vi "Insight_X-axis_OCT.vi"(6 "Index of Refraction":dbl=1.0 format="%_3g", 8 "error in (no error)":errorcluster, 10 "Size of FFT":u32, 11 "Spacing (GHz)":dbl=0.1 format="%_6g") -> (0 "error out":errorcluster, 1 "X-resolution (mm)":dbl, 2 "X-axis":dbl[](array[numeric]))   [LabVIEW 2011]
doc: "Insight Photonic Solutions\n\nThis VI calculates the X-axis for an OCT measurement.\n\nINPUTS\nSize of FFT - This is the size of the two-sided FFT. This may or may not be padded.\nSpacing (GHz) - Optical Frequency Spacing between samples of the measurement.\nIndex of Refraction - Default is 1.\n\nOUTPUTS\nX-resolution - spatial step between points, in millimeters.\nX-axis - Array containing the spatial axis for the OCT measurement.\n\nver 1.0 - original release"
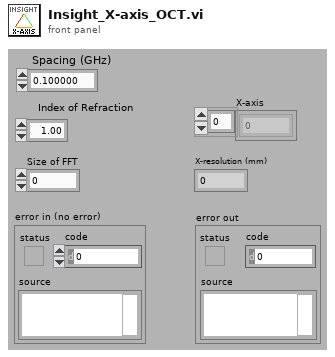
[diagram p1: front panel]
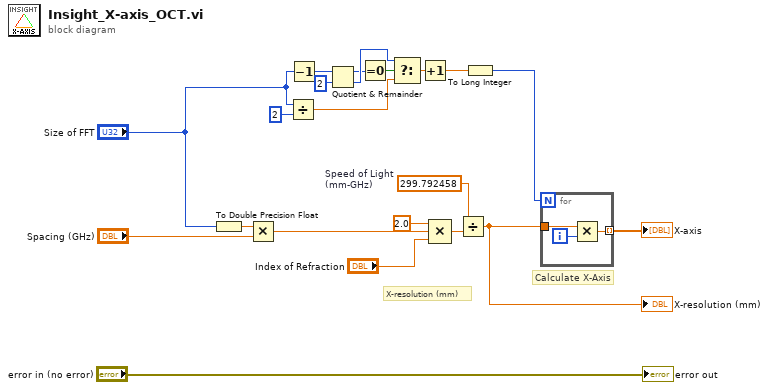
[diagram p0: block diagram]
diagram:
  w17 = 299.792458  # Speed of Light  (mm-GHz)
  # "X-resolution (mm)"
  # "Calculate X-Axis"
  n1 = To Double Precision Float(number="Size of FFT") -> (double precision float=w12:dbl)
  n2 = Multiply(x=w12, y="Spacing (GHz)") -> (x*y=w15:dbl)
  n3 = Divide(x="Size of FFT", y=2) -> (x/y=w11:dbl)
  n4 = Decrement(x="Size of FFT") -> (x-1=w5:u32)
  n5 = Quotient & Remainder(x=w5, y=2) -> (x-y*floor(x/y)=w7:u32, floor(x/y)=w9:u32)
  n6 = Equal To 0?(x=w7) -> (x = 0?=w8:bool)
  n7 = Select(t=w9, s=w8, f=w11) -> (s? t:f=w3:dbl)
  n8 = Increment(x=w3) -> (x+1=w2:dbl)
  n9 = Compound Arithmetic op=MULTIPLY(2.0, w15, "Index of Refraction") -> (w18:dbl)
  n10 = Divide(x=w17, y=w18) -> (x/y=w16:dbl)
  "X-resolution (mm)" <- w16
  n11 = To Long Integer(number=w2) -> (32bit integer=w1:i32)
  n12 = for {
    N: w1 -> [_]
    tunnel: w16 -> [w23]
    tunnel: [w22] -> w14 mode=indexing
    i -> [w24]
    n13 = Multiply(x=w23, y=w24) -> (x*y=w22:dbl)
  }
  "X-axis" <- w14
  "error out" <- "error in (no error)"
